vi "Limit AO Amplitude.vi"(8 "error in (no error)":errorcluster, 11 "Instrument.DAQ":refnum<class "Instrument.DAQ.lvclass">) -> (0 "error out":errorcluster, 3 "Instrument.DAQ out":refnum<class "Instrument.DAQ.lvclass">)   [LabVIEW 2019, in "Instrument.Lockin.lvlib" / "Instrument.DAQ.lvclass"]
uses:
  Instrument.DAQ.lvclass
  Instrument.DAQ.lvclass/Instrument.DAQ.ctl
panel:
  # "limit Amp"
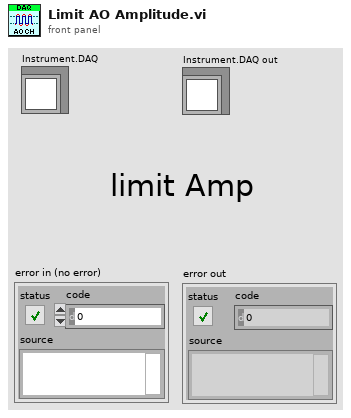
[diagram p1: front panel]
types:
  T1 = typedef "Instrument.Lockin.lvlib/Instrument.DAQ.lvclass/AO.Channel--Cluster--Array.ctl" = T2[]
  T2 = typedef "Instrument.Lockin.lvlib/Instrument.DAQ.lvclass/AO.Channel--Cluster.ctl" = cluster{"Enable?":bool, "Channel":i32, "Amplitude":dbl, "Offset":dbl, "Frequency":dbl, "Phase":dbl, "Function":T3, "Sweeping?":bool, "Limit AC":bool, "Limit DC?":bool, "Duty Cycle":bool}
  T3 = typedef "Instrument.Lockin.lvlib/Instrument.DAQ.lvclass/AO.Channel.Function--Enum.ctl" = enum16{"sine", "square", "triangle", "saw"}
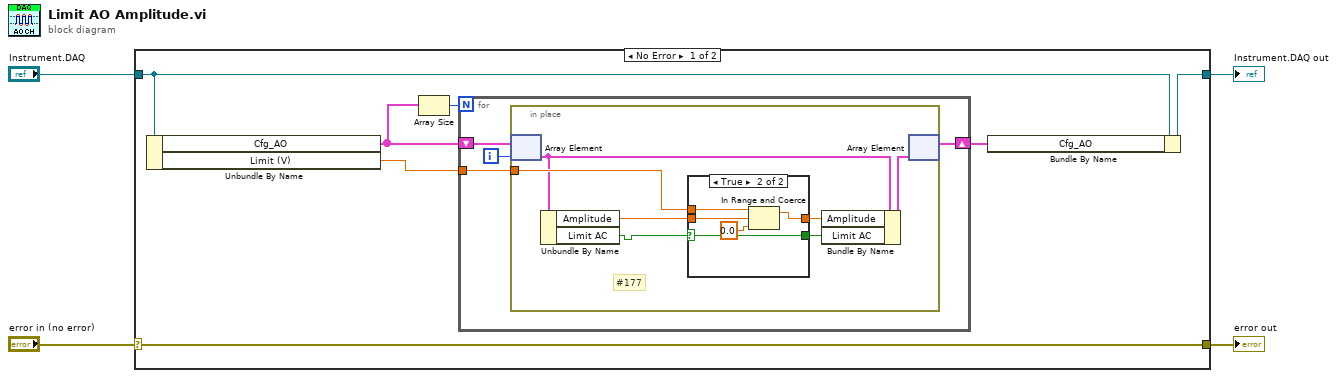
[diagram p0: block diagram]
diagram:
  n1 = case shown="No Error" "error in (no error)" {
    selector: "error in (no error)" -> [w8 w31]
    tunnel: [w11 w30] -> w4
    tunnel: "Instrument.DAQ" -> [w10 w30]
    tunnel: [w8 w31] -> w2
    frame No Error {
      n2 = Unbundle By Name(w10) -> ("Cfg_AO"=w6:T1, "Limit (V)"=w5:dbl)
      n3 = Array Size(array=w6) -> (size(s)=w7:i32)
      n4 = for {
        N: w7 -> [_]
        tunnel: w5 -> [w15]
        shift-right: [w13] -> w9
        shift-left: w6 -> [w14]
        i -> [w12]
        n5 = in-place {
          in-place-border: w15 -> [w19]
          # "#177"
          n6 = in-place-array #1(w14, w12) -> (w18:T2)
          n7 = Unbundle By Name(w18) -> ("Amplitude"=w22:dbl, "Limit AC"=w16:bool)
          n8 = case shown="True" w16 {
            selector: w16 -> [w23 w26]
            tunnel: w22 -> [w24 w28]
            tunnel: w19 -> [_ w25]
            tunnel: [w24 w27] -> w21
            tunnel: [w23 w26] -> w20
            frame False {
            }
            frame True {
              n9 = In Range and Coerce(upper limit=w25, x=w28, lower limit=0.0) -> (coerced(x)=w27:dbl)  [unwired: 1 out]
            }
          }
          n10 = Bundle By Name(cluster=w18, "Amplitude"=w21, "Limit AC"=w20) -> (w17:T2)
          n11 = in-place-array #1(w17) -> (w13:T1)  [unwired: 1 out]
        }
      }
      n12 = Bundle By Name(cluster=w10, "Cfg_AO"=w9) -> (w11:refnum<class "Instrument.DAQ.lvclass">)
    }
    frame Error {
    }
  }
  "Instrument.DAQ out" <- w4
  "error out" <- w2
